vi "Main Page.vi"(8 "error in (no error)":errorcluster, 11 "Node Ptr":T3 format="%.0x") -> (0 "error out":errorcluster)   [LabVIEW 2015, in "NI 9759 RevB Custom Device.lvlib"]
uses:
  NI 9759 RevB Custom Device.lvlib
  <vilib>/NI Veristand/Custom Device API/Custom Device Item Ref.ctl
  System.Windows.Forms
  <vilib>/NI Veristand/Custom Device API/Dependent File Optional Info.ctl
  Shared/9759 Properties.vi
  <vilib>/NI Veristand/Custom Device API/Set Item Property (Boolean).vi
  Shared/9759 Constants and GUIDs.vi
  <vilib>/NI Veristand/Custom Device API/Get Item Property (String).vi
  <vilib>/NI Veristand/Custom Device API/Get Item Property (I32).vi
  <vilib>/NI Veristand/Custom Device API/Get Item Property (Dependent File).vi
  <vilib>/NI Veristand/Custom Device API/Get Item Property (U16).vi
  <vilib>/NI Veristand/Custom Device API/Set Item Property (String).vi
  <vilib>/NI Veristand/Custom Device API/Set Item Property (U16).vi
  <vilib>/NI Veristand/Custom Device API/Set Item Property (I32).vi
  <vilib>/NI Veristand/Custom Device API/Set Item Property (Dependent File).vi
  <vilib>/NI VeriStand/Custom Device API/Custom Device API.lvlib
panel:
  in  "Position Calibrations":T1(array[cluster])
  in  "Control Calibrations":T2(array[cluster]) {"ThetaLH (deg)" format="%.3f"; "ULHLag (sec)" format="%.3f"; "USLag (sec)" format="%.3f"; "TLead (sec)" format="%.3f"; "TLag (sec)" format="%.3f"}
  in  "Header 4":cluster{"Section Name":string}={"Section Name"="Throttle Calibration Settings"}
  in  "Header 3":cluster{"Section Name":string}={"Section Name"="Bitfile Setup"}
  in  "Header 2":cluster{"Section Name":string}={"Section Name"="FPGA Target Setup"}
  in  "FPGA Resource":string="RIO0"
  in  "IP Address":string
  in  "FPGA Location":enum16{"Local", "Remote"}(ring)
  in  "Bitfile Path":path
  in  "CPU":i32=-2
  out "Device Address":string="RIO0"
  in  "Rate decimation":i32=1 min=1
  in  "Execution priority":enum16{"Low", "Medium", "High"}(ring)=enum."Medium"
  out "CD Version":string caption="Custom Device Version"
  in  "Header":cluster{"Section Name":string}={"Section Name"="Real-Time Target Setup"}
  in  "Device Name":string
  # "(-2: automatic)"
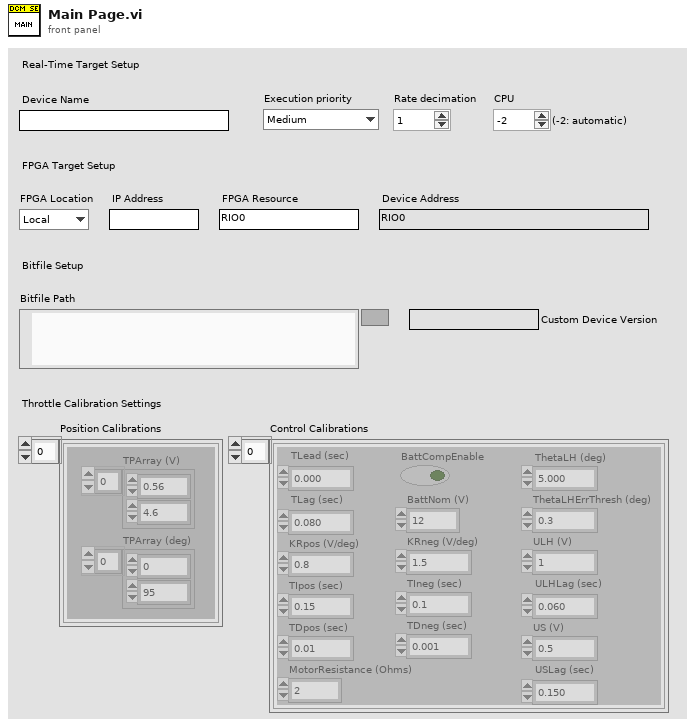
[diagram p1: front panel]
types:
  T1 = cluster{"TPArray (V)":sgl[], "TPArray (deg)":sgl[]}[]
  T2 = cluster{"TLead (sec)":sgl, "TLag (sec)":sgl, "KRpos (V/deg)":sgl, "TIpos (sec)":sgl, "TDpos (sec)":sgl, "KRneg (V/deg)":sgl, "TIneg (sec)":sgl, "TDneg (sec)":sgl, "ThetaLHErrThresh (deg)":sgl, "ULH (V)":sgl, "ULHLag (sec)":sgl, "US (V)":sgl, "USLag (sec)":sgl, "ThetaLH (deg)":sgl, "MotorResistance (Ohms)":sgl, "BattNom (V)":sgl, "BattCompEnable":bool}[]
  T3 = typedef "Custom Device API.lvlib/Custom Device Item Ref.ctl" = u64
  T4 = typedef "Custom Device API.lvlib/Custom Device Timed Loop Priority.ctl" = enum32{"Low", "Medium", "High"}
  T5 = typedef "Custom Device API.lvlib/Custom Device Item Info.ctl" = cluster{"Name":string, "Is Channel":bool, "GUID":string, "Is Waveform":bool}
  T6 = enum8{"Enabled", "Disabled", "Disabled and Grayed Out"}
  T7 = typedef "Custom Device API.lvlib/Dependent File Optional Info.ctl" = cluster{"Version":string, "RTDestination":path, "ForceDownload":bool, "SupportedTarget":string, "MD5":string}
  T8 = typedef "Custom Device API.lvlib/Custom Device Commands.ctl" = enum16{"Default", "Item renamed", "Shutdown", "Dynamic button pressed"}
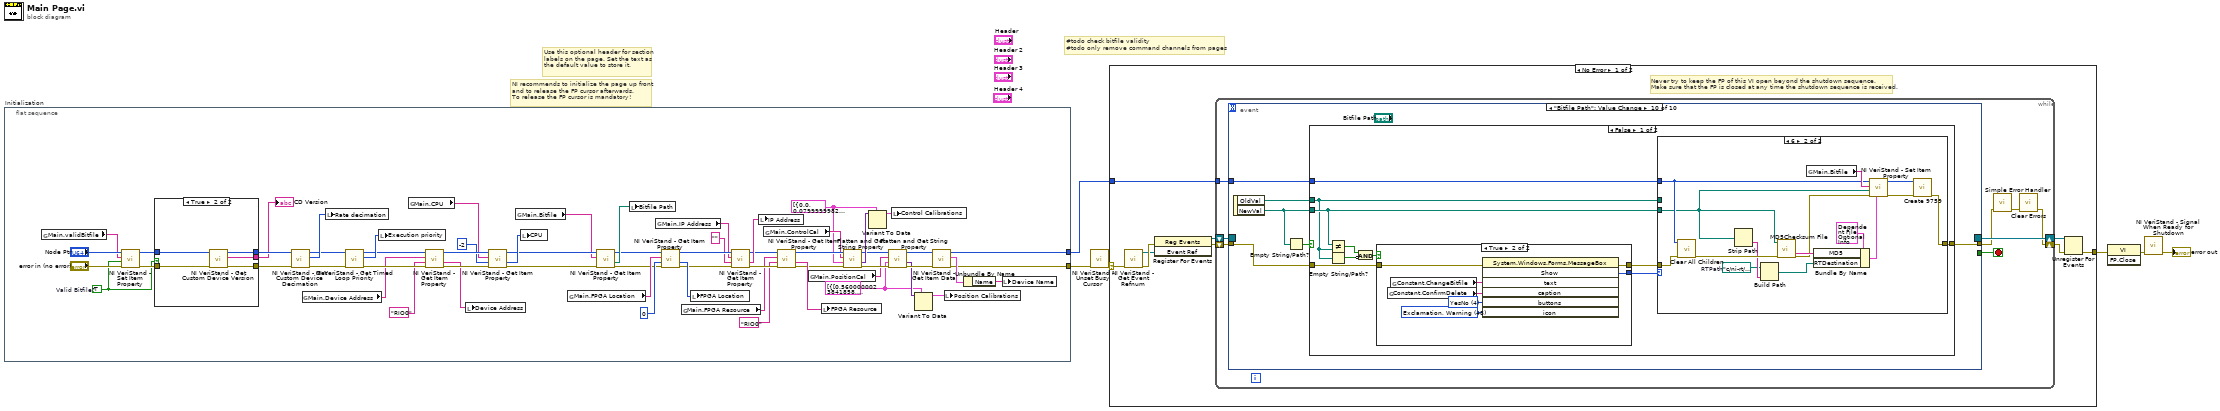
[diagram p0: block diagram]
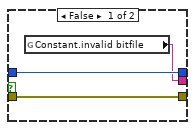
[diagram p2: hidden frame]
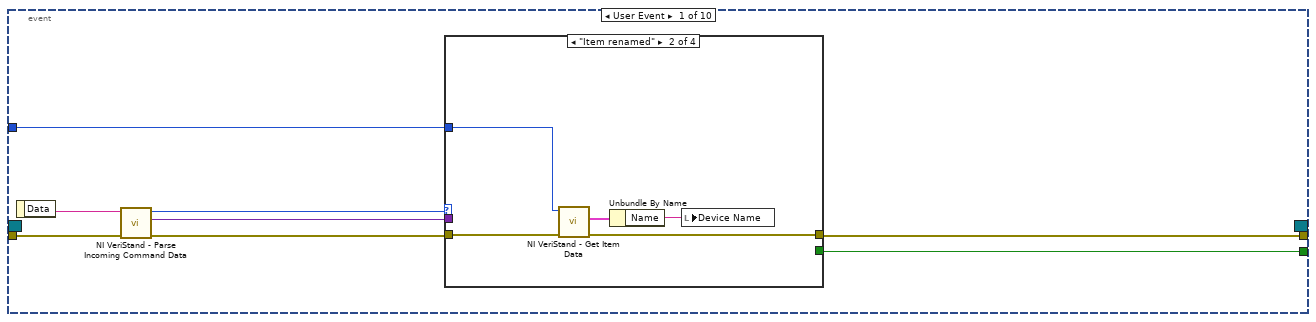
[diagram p3: hidden frame]
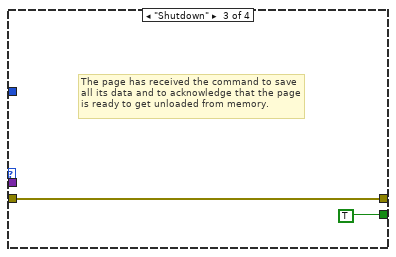
[diagram p5: hidden frame]
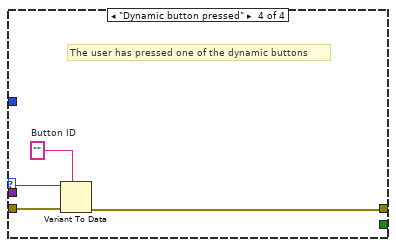
[diagram p6: hidden frame]
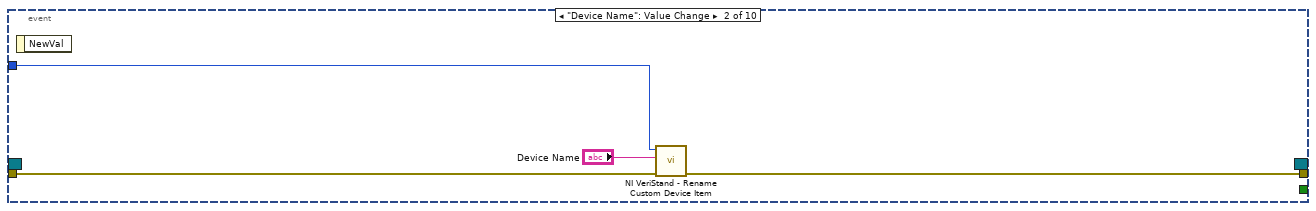
[diagram p7: hidden frame]
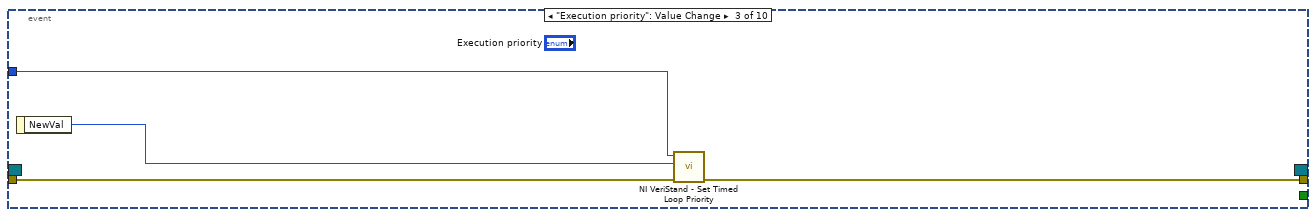
[diagram p8: hidden frame]
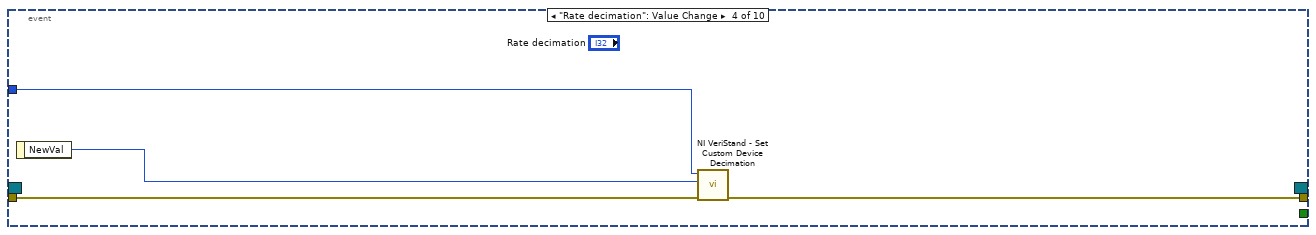
[diagram p9: hidden frame]
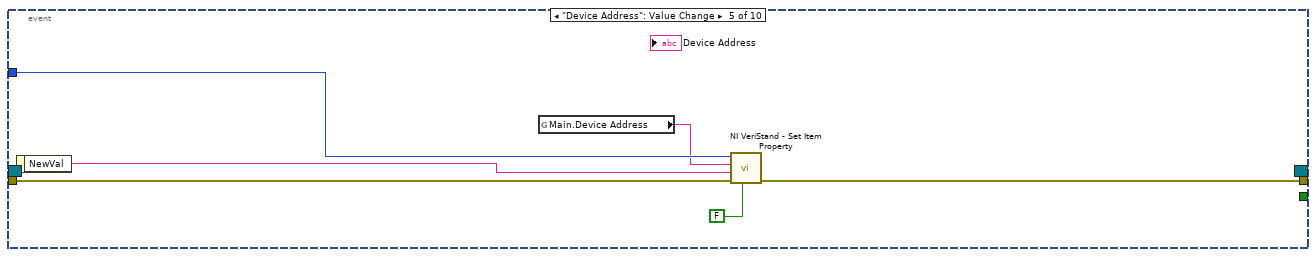
[diagram p10: hidden frame]
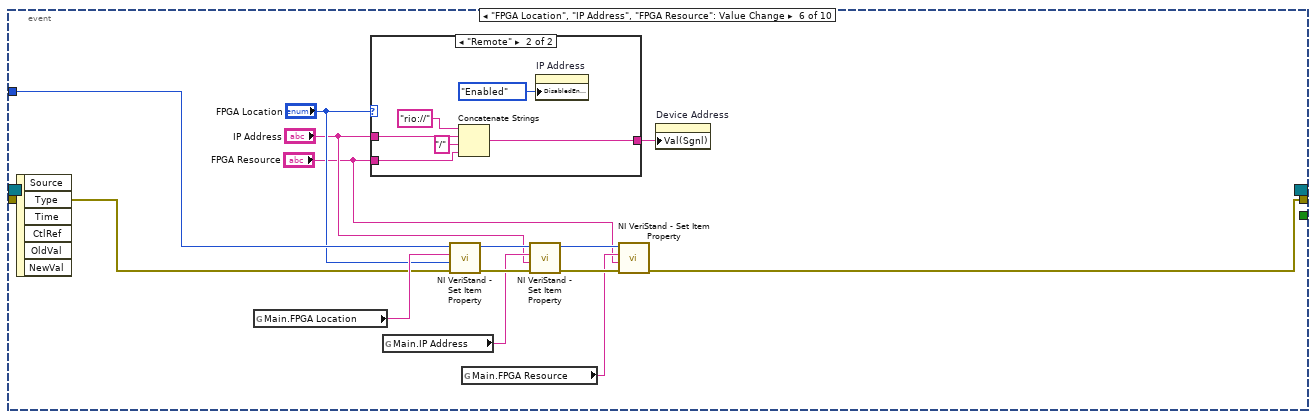
[diagram p11: hidden frame]
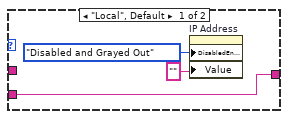
[diagram p12: hidden frame]
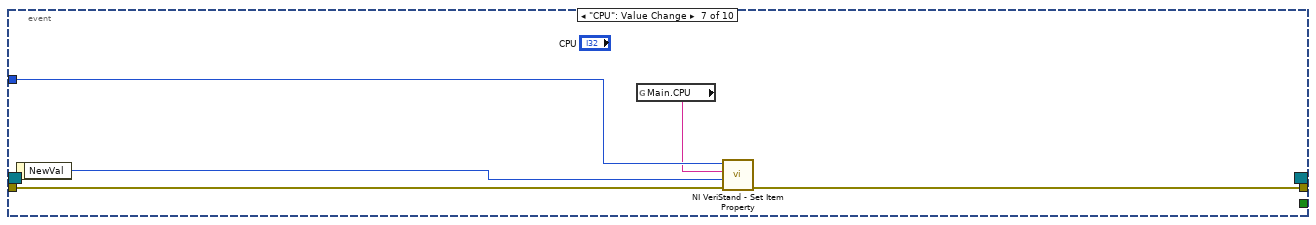
[diagram p13: hidden frame]
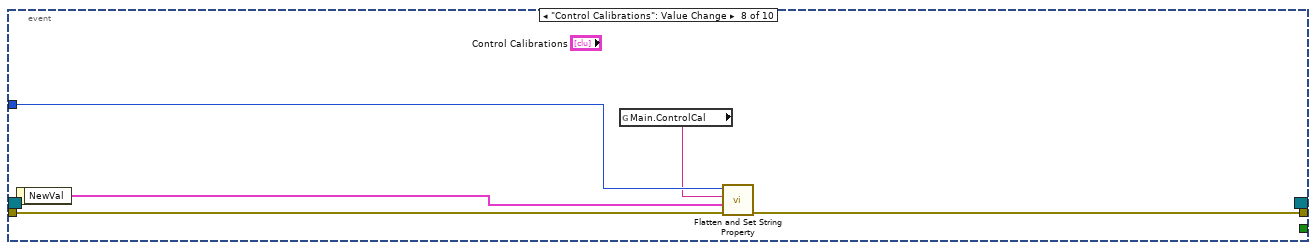
[diagram p14: hidden frame]
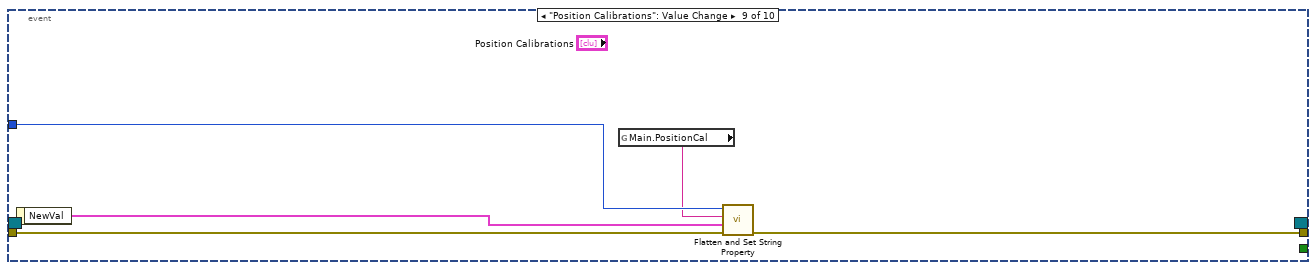
[diagram p15: hidden frame]
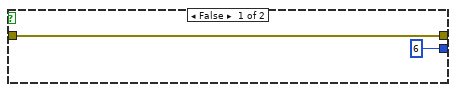
[diagram p16: hidden frame]
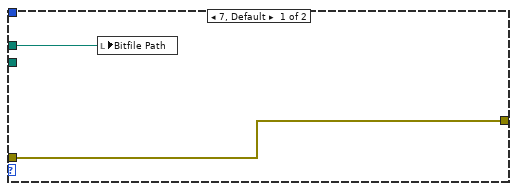
[diagram p17: hidden frame]
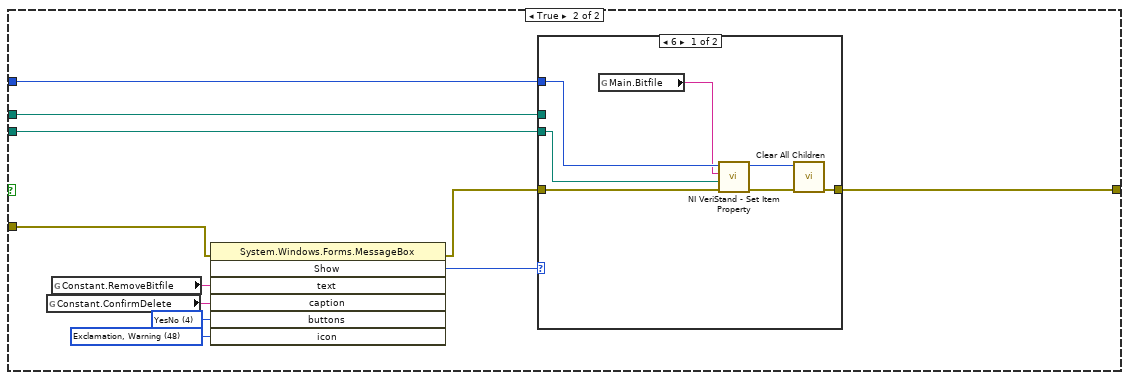
[diagram p18: hidden frame]
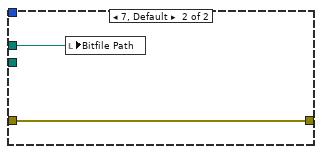
[diagram p19: hidden frame]
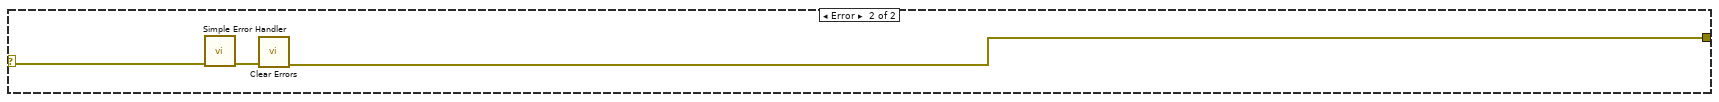
[diagram p20: hidden frame]
diagram:
  # "#todo check bitfile validity\n#todo only remove command channels from pages"
  # "Use this optional header for section labels on the page. Set the text as the default value to store it."
  # "NI recommends to initialize the page up front\nand to release the FP cursor afterwards.\nTo release the FP cursor is mandatory!"
  n1 = flat-sequence "Initialization" {
    tunnel: [w38] -> w2
    tunnel: [w39] -> w1
    frame #0 {
      w7 = T2 [{"TLead (sec)"=0.0, "TLag (sec)"=0.08, "KRpos (V/deg)"=0.8, "TIpos (sec)"=0.15, "TDpos (sec)"=0.01, "KRneg (V/deg)"=1.5, "TIneg (sec)"=0.1, "TDneg (sec)"=0.001, "ThetaLHErrThresh (deg)"=0.3, "ULH (V)"=1.0, "ULHLag (sec)"=0.06, "US (V)"=0.5, "USLag (sec)"=0.15, "ThetaLH (deg)"=5.0, "MotorResistance (Ohms)"=2.0, "BattNom (V)"=12.0, "BattCompEnable"=FALSE}, {"TLead (sec)"=0.0, "TLag (sec)"=0.08, "KRpos (V/deg)"=0.8, "TIpos (sec)"=0.15, "TDpos (sec)"=0.01, "KRneg (V/deg)"=1.5, "TIneg (sec)"=0.1, "TDneg (sec)"=0.001, "ThetaLHErrThresh (deg)"=0.3, "ULH (V)"=1.0, "ULHLag (sec)"=0.06, "US (V)"=0.5, "USLag (sec)"=0.15, "ThetaLH (deg)"=5.0, "MotorResistance (Ohms)"=2.0, "BattNom (V)"=12.0, "BattCompEnable"=FALSE}]
      w8 = T1 [{"TPArray (V)"=[0.56, 4.6], "TPArray (deg)"=[0.0, 95.0]}, {"TPArray (V)"=[0.56, 4.6], "TPArray (deg)"=[0.0, 95.0]}]
      w44 = TRUE  # Valid Bitfile?
      n2 = global read "9759 Properties.vi" "Main.validBitfile"() -> (w49:string)
      n3 = call-poly <vilib>:"NI VeriStand - Set Item Property.vi"("error in (no error)"="error in (no error)", "Value"=w44, "Property Name"=w49, "Item Ref in"="Node Ptr") -> ("error out"=w47:errorcluster, "Item Ref out"=w48:T3)  [unwired: 5 in, 1 out]
      n4 = case shown="True" w44 {
        tunnel: [w68 w74] -> w63
        tunnel: [w69 w73] -> w61
        tunnel: w48 -> [w69 w72]
        tunnel: w47 -> [w68 w71]
        tunnel: [w67 w70] -> w46
        frame False {
          n5 = global read "9759 Constants and GUIDs.vi" "Constant.invalid bitfile"() -> (w67:string)
        }
        frame True {
          n6 = call <vilib>:"NI VeriStand - Get Custom Device Version.vi"("error in (no error)"=w71, "Device Ref in"=w72) -> ("error out"=w74:errorcluster, "Value"=w70:string, "Device Ref out"=w73:T3)  [unwired: 7 in]
        }
      }
      "CD Version" <- w46
      n7 = call <vilib>:"NI VeriStand - Get Custom Device Decimation.vi"("error in (no error)"=w63, "Device Ref in"=w61) -> ("error out"=w62:errorcluster, "Decimation"=w60:i32, "Device Ref out"=w58:T3)  [unwired: 7 in]
      n8 = global read "9759 Properties.vi" "Main.Device Address"() -> (w20:string)
      n9 = local write "Rate decimation"(w60) -> ()
      n10 = call <vilib>:"NI VeriStand - Get Timed Loop Priority.vi"("error in (no error)"=w62, "Device Ref in"=w58) -> ("error out"=w59:errorcluster, "Priority"=w57:T4, "Device Ref out"=w55:T3)  [unwired: 7 in]
      n11 = local write "Execution priority"(w57) -> ()
      n12 = global read "9759 Properties.vi" "Main.CPU"() -> (w45:string)
      n13 = call-poly <vilib>:"NI VeriStand - Get Item Property.vi"("error in (no error)"=w59, "Default Value"="RIO0", "Property Name"=w20, "Item Ref in"=w55) -> ("error out"=w56:errorcluster, "Value"=w37:string, "Item Ref out"=w52:T3)  [unwired: 4 in, 1 out]
      n14 = local write "Device Address"(w37) -> ()
      n15 = call-poly <vilib>:"NI VeriStand - Get Item Property.vi"("error in (no error)"=w56, "Default Value"=-2, "Property Name"=w45, "Item Ref in"=w52) -> ("error out"=w42:errorcluster, "Value"=w50:i32, "Item Ref out"=w43:T3)  [unwired: 4 in, 1 out]
      n16 = global read "9759 Properties.vi" "Main.Bitfile"() -> (w41:string)
      n17 = local write "CPU"(w50) -> ()
      n18 = global read "9759 Properties.vi" "Main.FPGA Location"() -> (w35:string)
      n19 = call-poly <vilib>:"NI VeriStand - Get Item Property.vi"("error in (no error)"=w42, "Property Name"=w41, "Item Ref in"=w43) -> ("error out"=w33:errorcluster, "Path"=w40:path, "Item Ref out"=w34:T3)  [unwired: 4 in, 2 out]
      n20 = local write "Bitfile Path"(w40) -> ()
      n21 = global read "9759 Properties.vi" "Main.IP Address"() -> (w29:string)
      n22 = call-poly <vilib>:"NI VeriStand - Get Item Property.vi"("error in (no error)"=w33, "Default Value"=u16 0, "Property Name"=w35, "Item Ref in"=w34) -> ("error out"=w30:errorcluster, "Value"=w32:u16, "Item Ref out"=w31:T3)  [unwired: 4 in, 1 out]
      n23 = global read "9759 Properties.vi" "Main.FPGA Resource"() -> (w22:string)
      n24 = local write "FPGA Location"(w32) -> ()
      n25 = call-poly <vilib>:"NI VeriStand - Get Item Property.vi"("error in (no error)"=w30, "Default Value"="", "Property Name"=w29, "Item Ref in"=w31) -> ("error out"=w25:errorcluster, "Value"=w27:string, "Item Ref out"=w26:T3)  [unwired: 4 in, 1 out]
      n26 = local write "IP Address"(w27) -> ()
      n27 = global read "9759 Properties.vi" "Main.ControlCal"() -> (w18:string)
      n28 = call-poly <vilib>:"NI VeriStand - Get Item Property.vi"("error in (no error)"=w25, "Default Value"="RIO0", "Property Name"=w22, "Item Ref in"=w26) -> ("error out"=w19:errorcluster, "Value"=w23:string, "Item Ref out"=w24:T3)  [unwired: 4 in, 1 out]
      n29 = global read "9759 Properties.vi" "Main.PositionCal"() -> (w11:string)
      n30 = local write "FPGA Resource"(w23) -> ()
      n31 = call "Flatten and Get String Property.vi"("error in (no error)"=w19, "Default Value"=w7, "Property Name"=w18, "Section Ref in"=w24) -> ("error out"=w12:errorcluster, "Value"=w17:variant, "Section Ref out"=w15:T3)  [unwired: 5 in]
      n32 = Variant To Data(type=w7, Variant=w17) -> (data=w16:T2)  [unwired: 1 in, 1 out]
      n33 = call "Flatten and Get String Property.vi"("error in (no error)"=w12, "Default Value"=w8, "Property Name"=w11, "Section Ref in"=w15) -> ("error out"=w13:errorcluster, "Value"=w10:variant, "Section Ref out"=w14:T3)  [unwired: 5 in]
      n34 = local write "Control Calibrations"(w16) -> ()
      n35 = Variant To Data(type=w8, Variant=w10) -> (data=w9:T1)  [unwired: 1 in, 1 out]
      n36 = call <vilib>:"NI VeriStand - Get Item Data.vi"("error in (no error)"=w13, "Item Ref in"=w14) -> ("error out"=w39:errorcluster, "Item Info"=w65:T5, "Item Ref out"=w38:T3)  [unwired: 7 out]
      n37 = local write "Position Calibrations"(w9) -> ()
      n38 = Unbundle By Name(w65) -> ("Name"=w64:string)
      n39 = local write "Device Name"(w64) -> ()
    }
  }
  n40 = call <vilib>:"NI VeriStand - Unset Busy Cursor.vi"("error in (no error)"=w1) -> ("error out"=w3:errorcluster)  [unwired: 10 out]
  n41 = case shown="No Error" w3 {
    selector: w3 -> [w76 w232]
    tunnel: [w80 w230] -> w6
    tunnel: w2 -> [w75 _]
    frame No Error {
      # "Never try to keep the FP of this VI open beyond the shutdown sequence.\nMake sure that the FP is closed at any time the shutdown sequence is received."
      n42 = call <vilib>:"NI VeriStand - Get Event Refnum.vi"("error in (no error)"=w76) -> ("error out"=w83:errorcluster, "Event Ref"=w79:refnum<user-event>)  [unwired: 9 out]
      n43 = register-events(error in=w83, w79) -> (reference out=w77:refnum<event-registration>, error out=w78:errorcluster)  [unwired: 1 in]
      n44 = while {
        shift-right: [w85] -> w81
        shift-left: w78 -> [w90]
        shift-right: [w91] -> w82
        shift-left: w77 -> [w89]
        tunnel: w75 -> [w84]
        stop <- w88 stop-if-true
        n45 = event shown="[9] \"Bitfile Path\": Value Change" {
          selector: w89 -> [_ _ _ _ _ _ _ _ _ _]
          dyn-events: [_ _ _ _ _ _ _ _ _ _] -> w91
          timeout: _ -> [_ _ _ _ _ _ _ _ _ _]
          tunnel: w90 -> [w99 w115 w119 w123 w129 w135 w157 w162 w167 w173]
          tunnel: [w95 _ _ _ _ _ _ _ _ _] -> w88
          tunnel: [w94 w114 w118 w122 w127 w134 w155 w160 w165 w172] -> w87
          tunnel: w84 -> [w92 w112 w116 w120 w125 w141 w154 w159 w164 w171]
          event User Event {
            n46 = event-data() -> ("Data"=w98:string)  [unwired: 1 out]
            n47 = call <vilib>:"NI VeriStand - Parse Incoming Command Data.vi"("error in (no error)"=w99, "Incoming data"=w98) -> ("error out"=w97:errorcluster, "Outgoing data"=w93:variant, "Action"=w96:T8)  [unwired: 7 out]
            n48 = case shown="\"Item renamed\"" w96 {
              tunnel: w97 -> [w100 w105 w106 w111]
              tunnel: [_ _ TRUE _] -> w95
              tunnel: [w100 w103 w106 w108] -> w94
              tunnel: w93 -> [_ _ _ w110]
              tunnel: w92 -> [_ w101 _ _]
              frame "Default", Default {
              }
              frame "Item renamed" {
                n49 = call <vilib>:"NI VeriStand - Get Item Data.vi"("error in (no error)"=w105, "Item Ref in"=w101) -> ("error out"=w103:errorcluster, "Item Info"=w104:T5)  [unwired: 8 out]
                n50 = Unbundle By Name(w104) -> ("Name"=w102:string)
                n51 = local write "Device Name"(w102) -> ()
              }
              frame "Shutdown" {
                # "The page has received the command to save all its data and to acknowledge that the page is ready to get unloaded from memory."
              }
              frame "Dynamic button pressed" {
                w109 = ""  # Button ID
                # "The user has pressed one of the dynamic buttons"
                n52 = Variant To Data(error in=w111, type=w109, Variant=w110) -> (error out=w108:errorcluster)  [unwired: 1 out]
              }
            }
          }
          event "Device Name": Value Change {
            n53 = event-data() -> ()  [unwired: 2 out]
            n54 = call <vilib>:"NI VeriStand - Rename Custom Device Item.vi"("error in (no error)"=w115, "New Name"="Device Name", "Item Ref in"=w112) -> ("error out"=w114:errorcluster)  [unwired: 1 in, 7 out]
          }
          event "Execution priority": Value Change {
            n55 = event-data() -> ("NewVal"=w117:enum16{"Low", "Medium", "High"})  [unwired: 1 out]
            n56 = call <vilib>:"NI VeriStand - Set Timed Loop Priority.vi"("error in (no error)"=w119, "Priority"=w117, "Device Ref in"=w116) -> ("error out"=w118:errorcluster)  [unwired: 7 in, 1 out]
          }
          event "Rate decimation": Value Change {
            n57 = event-data() -> ("NewVal"=w121:i32)  [unwired: 1 out]
            n58 = call <vilib>:"NI VeriStand - Set Custom Device Decimation.vi"("error in (no error)"=w123, "Decimation"=w121, "Device Ref in"=w120) -> ("error out"=w122:errorcluster)  [unwired: 7 in, 1 out]
          }
          event "Device Address": Value Change {
            n59 = event-data() -> ("NewVal"=w128:string)  [unwired: 1 out]
            n60 = global read "9759 Properties.vi" "Main.Device Address"() -> (w124:string)
            n61 = call-poly <vilib>:"NI VeriStand - Set Item Property.vi"("Binary String (T)"=FALSE, "error in (no error)"=w129, "Value"=w128, "Property Name"=w124, "Item Ref in"=w125) -> ("error out"=w127:errorcluster)  [unwired: 4 in, 2 out]
          }
          event "FPGA Location", "IP Address", "FPGA Resource": Value Change {
            n62 = event-data() -> ()  [unwired: 7 out]
            n63 = global read "9759 Properties.vi" "Main.FPGA Location"() -> (w142:string)
            n64 = case shown="\"Remote\"" "FPGA Location" {
              tunnel: "IP Address" -> [_ w151]
              tunnel: "FPGA Resource" -> [w146 w150]
              tunnel: [w146 w148] -> w143
              frame "Local", Default {
                n65 = property on="IP Address" class="Str"("DisabledEnum"=T6."Disabled and Grayed Out" ("Disabled"), "Value"="" ("IP Address")) -> ()  [unwired: 2 in, 2 out]
              }
              frame "Remote" {
                n66 = Concatenate Strings("rio://", w151, "/" ("string"), w150) -> (w148:string)
                n67 = property on="IP Address" class="Str"("DisabledEnum"=T6."Enabled" ("Disabled")) -> ()  [unwired: 2 in, 2 out]
              }
            }
            n68 = global read "9759 Properties.vi" "Main.IP Address"() -> (w132:string)
            n69 = call-poly <vilib>:"NI VeriStand - Set Item Property.vi"("error in (no error)"=w135, "Value"="FPGA Location", "Property Name"=w142, "Item Ref in"=w141) -> ("error out"=w138:errorcluster, "Item Ref out"=w139:T3)  [unwired: 5 in, 1 out]
            n70 = global read "9759 Properties.vi" "Main.FPGA Resource"() -> (w133:string)
            n71 = call-poly <vilib>:"NI VeriStand - Set Item Property.vi"("error in (no error)"=w138, "Value"="IP Address", "Property Name"=w132, "Item Ref in"=w139) -> ("error out"=w137:errorcluster, "Item Ref out"=w136:T3)  [unwired: 5 in, 1 out]
            n72 = call-poly <vilib>:"NI VeriStand - Set Item Property.vi"("error in (no error)"=w137, "Value"="FPGA Resource", "Property Name"=w133, "Item Ref in"=w136) -> ("error out"=w134:errorcluster)  [unwired: 5 in, 2 out]
            n73 = property on="Device Address" class="Str"("Val(Sgnl)"=w143) -> ()  [unwired: 2 in, 2 out]
          }
          event "CPU": Value Change {
            n74 = event-data() -> ("NewVal"=w156:i32)  [unwired: 1 out]
            n75 = global read "9759 Properties.vi" "Main.CPU"() -> (w153:string)
            n76 = call-poly <vilib>:"NI VeriStand - Set Item Property.vi"("error in (no error)"=w157, "Value"=w156, "Property Name"=w153, "Item Ref in"=w154) -> ("error out"=w155:errorcluster)  [unwired: 5 in, 2 out]
          }
          event "Control Calibrations": Value Change {
            n77 = event-data() -> ("NewVal"=w161:T2)  [unwired: 1 out]
            n78 = global read "9759 Properties.vi" "Main.ControlCal"() -> (w158:string)
            n79 = call "Flatten and Set String Property.vi"("error in (no error)"=w162, "Value"=w161, "Property Name"=w158, "Section Ref in"=w159) -> ("error out"=w160:errorcluster)  [unwired: 6 in, 1 out]
          }
          event "Position Calibrations": Value Change {
            n80 = event-data() -> ("NewVal"=w166:T1)  [unwired: 1 out]
            n81 = global read "9759 Properties.vi" "Main.PositionCal"() -> (w163:string)
            n82 = call "Flatten and Set String Property.vi"("error in (no error)"=w167, "Value"=w166, "Property Name"=w163, "Section Ref in"=w164) -> ("error out"=w165:errorcluster)  [unwired: 6 in, 1 out]
          }
          event "Bitfile Path": Value Change {
            n83 = event-data() -> ("OldVal"=w168:path, "NewVal"=w169:path)  [unwired: 1 out]
            n84 = Empty String/Path?(string/path=w169) -> (empty?=w170:bool)
            n85 = case shown="False" w170 {
              tunnel: w173 -> [w183 w216]
              tunnel: [w182 w212] -> w172
              tunnel: w171 -> [w181 w211]
              tunnel: w169 -> [w175 w210]
              tunnel: w168 -> [w174 w214]
              frame False {
                n86 = Not Equal?(x=w175, y=w174) -> (x != y?=w176:bool)
                n87 = Empty String/Path?(string/path=w174) -> (empty?=w178:bool)
                n88 = Compound Arithmetic op=AND(w176, invert w178) -> (w177:bool)
                n89 = case shown="True" w177 {
                  tunnel: w183 -> [w185 w190]
                  tunnel: [6 ("Show") w189] -> w180
                  tunnel: [w185 w188] -> w179
                  frame False {
                  }
                  frame True {
                    w192 = 4 items=["OK", "OKCancel", "AbortRetryIgnore", "YesNoCancel", "YesNo", "RetryCancel"] ("buttons")
                    w191 = 48 items=["None"=0, "Hand, Error, Stop"=16, "Question"=32, "Exclamation, Warning"=48, "Asterisk, Information"=64] ("icon")
                    n90 = global read "9759 Constants and GUIDs.vi" "Constant.ConfirmDelete"() -> (w186:string)
                    n91 = global read "9759 Constants and GUIDs.vi" "Constant.ChangeBitfile"() -> (w187:string)
                    n92 = invoke class="System.Windows.Forms.MessageBox" method="Show"(error in=w190, "text"=w187, "caption"=w186, "buttons"=w192, "icon"=w191) -> (error out=w188:errorcluster, "Show"=w189:i32)  [unwired: 2 in, 5 out]
                  }
                }
                n93 = case shown="6" w180 {
                  tunnel: w179 -> [w194 w209]
                  tunnel: [w194 w206] -> w182
                  tunnel: w181 -> [_ w207]
                  tunnel: w175 -> [_ w196]
                  tunnel: w174 -> [w193 _]
                  frame 7, Default {
                    n94 = local write "Bitfile Path"(w193) -> ()
                  }
                  frame 6 {
                    w195 = path "c:/ni-rt/NIVeriStand/Custom Devices/bitfiles"  # RTPath
                    n95 = call "Clear All Children.vi"("error in (no error)"=w209, "Item Ref in"=w207) -> ("error out"=w202:errorcluster)  [unwired: 8 in, 1 out]
                    n96 = Strip Path(path=w196) -> (name=w197:string)  [unwired: 1 out]
                    n97 = Build Path(base path=w195, name or relative path=w197) -> (appended path=w198:path)
                    n98 = call <vilib>:"MD5Checksum File.vi"("error in (no error)"=w202, "Path"=w196) -> ("error out"=w201:errorcluster, "MD5 message-digest"=w204:string)  [unwired: 8 in]
                    n99 = global read "9759 Properties.vi" "Main.Bitfile"() -> (w208:string)
                    n100 = Bundle By Name(cluster=T7 {"Version"="1.0", "RTDestination"=path "home/lvuser/natinst/NIVeriStand/Custom Devices/DCM-2116", "ForceDownload"=FALSE, "SupportedTarget"="All", "MD5"=""} ("OptionalInfo"), "MD5"=w204, "RTDestination"=w198) -> (w203:T7)
                    n101 = call-poly <vilib>:"NI VeriStand - Set Item Property.vi"("OptionalInfo"=w203, "error in (no error)"=w201, "Path"=w196, "Property Name"=w208, "Item Ref in"=w207) -> ("error out"=w199:errorcluster, "Item Ref out"=w200:T3)  [unwired: 4 in, 1 out]
                    n102 = call "Create 9759.vi"("error in (no error)"=w199, "Section Ptr"=w200) -> ("error out"=w206:errorcluster)  [unwired: 8 in, 1 out]
                  }
                }
              }
              frame True {
                w220 = 4 items=["OK", "OKCancel", "AbortRetryIgnore", "YesNoCancel", "YesNo", "RetryCancel"] ("buttons")
                w219 = 48 items=["None"=0, "Hand, Error, Stop"=16, "Question"=32, "Exclamation, Warning"=48, "Asterisk, Information"=64] ("icon")
                n103 = global read "9759 Constants and GUIDs.vi" "Constant.ConfirmDelete"() -> (w217:string)
                n104 = global read "9759 Constants and GUIDs.vi" "Constant.RemoveBitfile"() -> (w218:string)
                n105 = invoke class="System.Windows.Forms.MessageBox" method="Show"(error in=w216, "text"=w218, "caption"=w217, "buttons"=w220, "icon"=w219) -> (error out=w213:errorcluster, "Show"=w215:i32)  [unwired: 2 in, 5 out]
                n106 = case shown="6" w215 {
                  tunnel: w214 -> [_ w229]
                  tunnel: w213 -> [w223 w228]
                  tunnel: [w227 w228] -> w212
                  tunnel: w211 -> [w225 _]
                  tunnel: w210 -> [w222 _]
                  frame 6 {
                    n107 = global read "9759 Properties.vi" "Main.Bitfile"() -> (w221:string)
                    n108 = call-poly <vilib>:"NI VeriStand - Set Item Property.vi"("error in (no error)"=w223, "Path"=w222, "Property Name"=w221, "Item Ref in"=w225) -> ("error out"=w224:errorcluster, "Item Ref out"=w226:T3)  [unwired: 5 in, 1 out]
                    n109 = call "Clear All Children.vi"("error in (no error)"=w224, "Item Ref in"=w226) -> ("error out"=w227:errorcluster)  [unwired: 8 in, 1 out]
                  }
                  frame 7, Default {
                    n110 = local write "Bitfile Path"(w229) -> ()
                  }
                }
              }
            }
          }
        }
        n111 = call <vilib>:"Simple Error Handler.vi"("error in (no error)"=w87) -> ("error out"=w86:errorcluster)  [unwired: 1 in, 7 out]
        n112 = call <vilib>:"Clear Errors.vi"("error in (no error)"=w86) -> ("error out"=w85:errorcluster)  [unwired: 1 in, 5 out]
      }
      n113 = Unregister For Events(event registration refnum=w82, error in=w81) -> (error out=w80:errorcluster)
    }
    frame Error {
      n114 = call <vilib>:"Simple Error Handler.vi"("error in (no error)"=w232) -> ("error out"=w231:errorcluster)  [unwired: 1 in, 7 out]
      n115 = call <vilib>:"Clear Errors.vi"("error in (no error)"=w231) -> ("error out"=w230:errorcluster)  [unwired: 1 in, 5 out]
    }
  }
  n116 = invoke class="VI" method="FP.Close"(error in=w6) -> (error out=w5:errorcluster)  [unwired: 2 in, 2 out]
  n117 = call <vilib>:"NI VeriStand - Signal When Ready for Shutdown.vi"("error in (no error)"=w5) -> ("error out"=→"error out":errorcluster)  [unwired: 10 out]
